vi "Enable Noise Floor Extensions.vi"(8 "error in (no error)":errorcluster, 10 "Enable Noise Floor Extensions (F: Disable)":bool, 11 "VISA resource name":refnum<visa-resource-name>) -> (0 "error out":errorcluster, 3 "VISA resource name out":refnum<visa-resource-name>)   [LabVIEW 2018, in "Agilent MXA Series.lvlib"]
doc: "Enable noise floor extensions function. \n\n<B>Note:</B>\n\nThis VI only applies to Agilent PXA series."
uses:
  Agilent MXA Series.lvlib
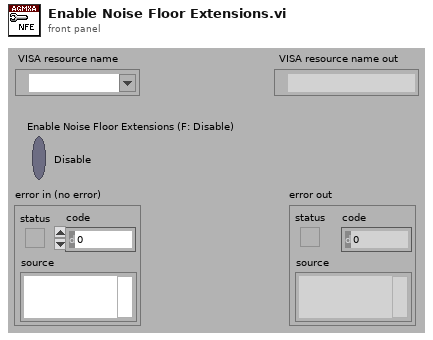
[diagram p1: front panel]
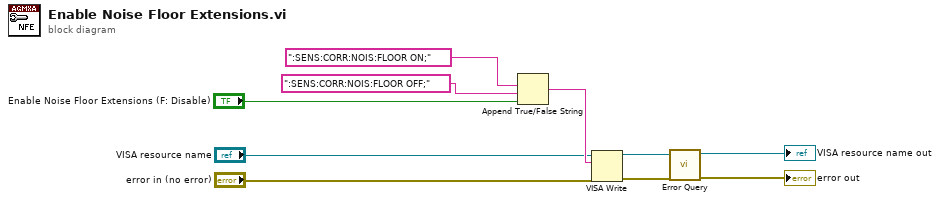
[diagram p0: block diagram]
diagram:
  n1 = Append True/False String(1:"Enable Noise Floor Extensions (F: Disable)", 2:":SENS:CORR:NOIS:FLOOR OFF;" ("false string"), 3:":SENS:CORR:NOIS:FLOOR ON;" ("true string")) -> (0:w6:string)  [unwired: 1 in]
  n2 = VISA Write(VISA resource name="VISA resource name", write buffer=w6, error in (no error)="error in (no error)") -> (VISA resource name out=w9:refnum<visa-resource-name>, error out=w10:errorcluster)  [unwired: 1 out]
  n3 = call "Error Query.vi"("error in (no error)"=w10, "VISA resource name"=w9) -> ("error out"=→"error out":errorcluster, "VISA resource name out"=→"VISA resource name out":refnum<visa-resource-name>)  [unwired: 6 in, 2 out]
